vi "Configure Trigger.vi"(8 "error in (no error)":errorcluster, 9 "Trigger Holdoff (0.00 sec)":dbl format="%.2p", 10 "Trigger Type (Edge)":string(combo)="Edge", 11 "VISA Resource Name":refnum<visa-resource-name>) -> (0 "error out":errorcluster, 3 "VISA Resource Name Out":refnum<visa-resource-name>)   [LabVIEW 2010, in "Tektronix TDS 3000 Series.lvlib"]
doc: "This function configures the common values of the trigger subsystem. These values are the trigger type and holdoff.\n\nWhen you call tktds3k Read Waveform or tktds3k Read Waveform Measurement, the oscilloscope waits for a trigger. You specify the type of trigger for which the oscilloscope waits with the Trigger Type control. \n\nIf the oscilloscope requires multiple waveform acquisitions to build a complete waveform, it waits for the length of time you specify with the Holdoff control to elapse since the previous trigger. The oscilloscope then waits for the next trigger. Once the oscilloscope acquires a complete waveform, it returns to the Idle state.\n\nNotes:\n\n(1) After you call this VI, you must call the trigger configuration function that corresponds to the Trigger Type you select to completely specify the trigger. For example, if you set the Trigger Type to Edge Trigger, you use the tktds3k Configure Edge Trigger Source VI to completely specify the trigger."
uses:
  <instrlib>/Tektronix TDS 3000 Series/Tektronix TDS 3000 Series.lvlib
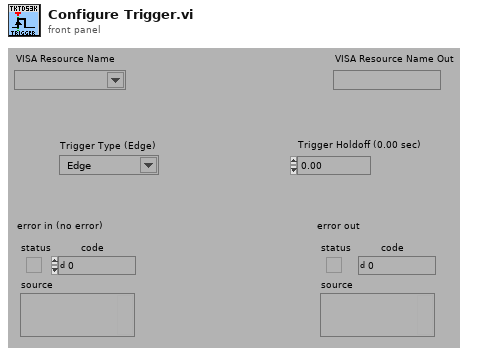
[diagram p1: front panel]
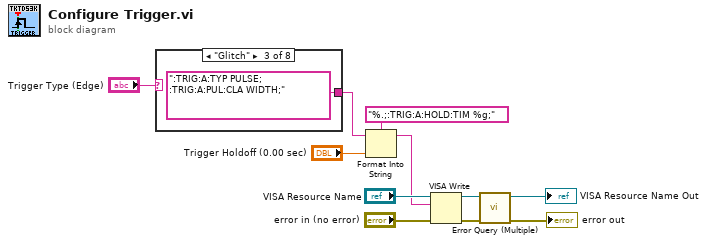
[diagram p0: block diagram]
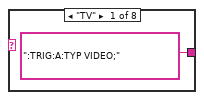
[diagram p2: hidden frame]
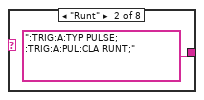
[diagram p3: hidden frame]
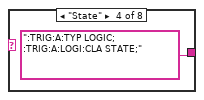
[diagram p4: hidden frame]
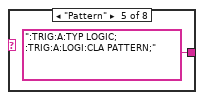
[diagram p5: hidden frame]
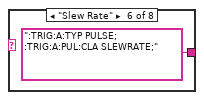
[diagram p6: hidden frame]
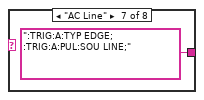
[diagram p7: hidden frame]
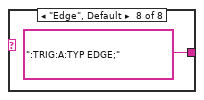
[diagram p8: hidden frame]
diagram:
  n1 = case shown="\"Glitch\"" "Trigger Type (Edge)" {
    tunnel: [":TRIG:A:TYP VIDEO;" ":TRIG:A:TYP PULSE; :TRIG:A:PUL:CLA RUNT;" ":TRIG:A:TYP PULSE; :TRIG:A:PUL:CLA WIDTH;" ":TRIG:A:TYP LOGIC; :TRIG:A:LOGI:CLA STATE;" ":TRIG:A:TYP LOGIC; :TRIG:A:LOGI:CLA PATTERN;" ":TRIG:A:TYP PULSE; :TRIG:A:PUL:CLA SLEWRATE;" ":TRIG:A:TYP EDGE; :TRIG:A:PUL:SOU LINE;" ":TRIG:A:TYP EDGE;"] -> w5
    frame "TV" {
    }
    frame "Runt" {
    }
    frame "Glitch" {
    }
    frame "State" {
    }
    frame "Pattern" {
    }
    frame "Slew Rate" {
    }
    frame "AC Line" {
    }
    frame "Edge", Default {
    }
  }
  n2 = Format Into String(format string="%.;:TRIG:A:HOLD:TIM %g;", initial string=w5, "Trigger Holdoff (0.00 sec)") -> (resulting string=w8:string)  [unwired: 1 in, 1 out]
  n3 = VISA Write(VISA resource name="VISA Resource Name", write buffer=w8, error in (no error)="error in (no error)") -> (VISA resource name out=w3:refnum<visa-resource-name>, error out=w4:errorcluster)  [unwired: 1 out]
  n4 = call <instrlib>:"Error Query (Multiple).vi"("error in (no error)"=w4, "VISA Resource Name"=w3) -> ("error out"=→"error out":errorcluster, "VISA Resource Name Out"=→"VISA Resource Name Out":refnum<visa-resource-name>)  [unwired: 6 in, 2 out]
